vi "תפריט מוכן.vi"() -> ()   [LabVIEW 2013]
panel:
  out "current time":timestamp format="%<%I:%M %p\n%x>T"
  in  "Exit to opening screen":bool
  in  "Production":bool
  in  "Warehouse":bool
  in  "Order Manegmrnt":bool
  # "Fider"
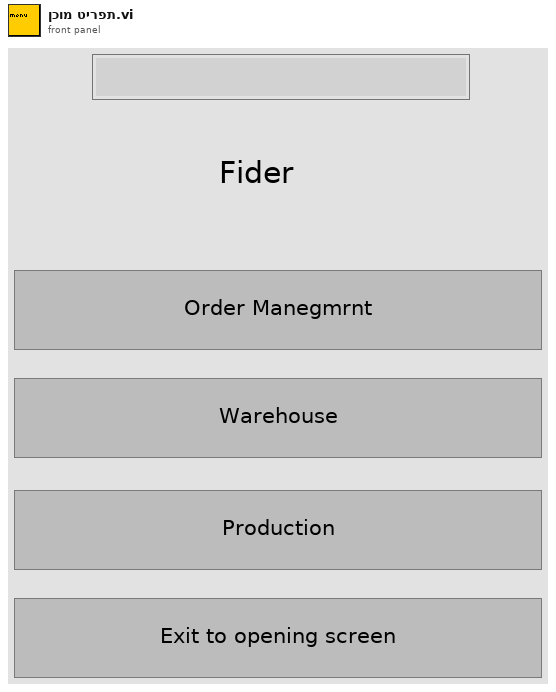
[diagram p1: front panel]
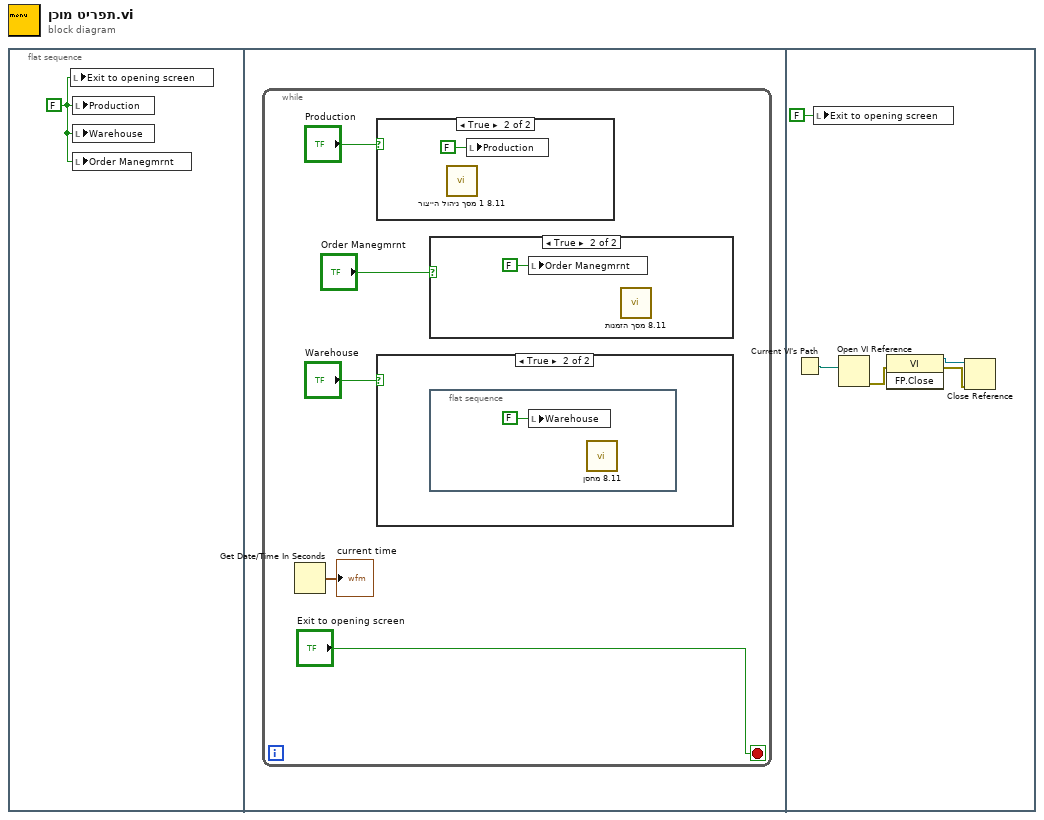
[diagram p0: block diagram]
diagram:
  n1 = flat-sequence {
    frame #0 {
      w1 = FALSE ("Exit to opening screen")
      n2 = local write "Exit to opening screen"(w1) -> ()
      n3 = local write "Production"(w1) -> ()
      n4 = local write "Warehouse"(w1) -> ()
      n5 = local write "Order Manegmrnt"(w1) -> ()
    }
    frame #1 {
      n6 = while {
        stop <- "Exit to opening screen" stop-if-true
        n7 = Get Date/Time In Seconds() -> (seconds since 1Jan1904=→"current time":timestamp)
        n8 = case shown="True" "Production" {
          frame False {
          }
          frame True {
            n9 = call "מסך ניהול הייצור 1 8.11.vi"() -> ()  [unwired: 1 in]
            n10 = local write "Production"(FALSE ("Production")) -> ()
          }
        }
        n11 = case shown="True" "Warehouse" {
          frame False {
          }
          frame True {
            n12 = flat-sequence {
              frame #0 {
                n13 = local write "Warehouse"(FALSE ("Warehouse")) -> ()
                n14 = call "מחסן 8.11.vi"() -> ()  [unwired: 1 in]
              }
            }
          }
        }
        n15 = case shown="True" "Order Manegmrnt" {
          frame False {
          }
          frame True {
            n16 = local write "Order Manegmrnt"(FALSE ("Order Manegmrnt")) -> ()
            n17 = call "מסך הזמנות 8.11.vi"() -> ()  [unwired: 1 in]
          }
        }
      }
    }
    frame #2 {
      n18 = Current VI's Path() -> (path=w13:path)
      n19 = local write "Exit to opening screen"(FALSE ("Exit to opening screen")) -> ()
      n20 = Open VI Reference(vi path=w13) -> (error out=w12:errorcluster)  [unwired: 5 in, 1 out]
      n21 = invoke class="VI" method="FP.Close"(error in=w12) -> (reference out=w10:refnum<vi>, error out=w11:errorcluster)  [unwired: 2 in, 1 out]
      n22 = Close Reference(reference=w10, error in (no error)=w11) -> ()  [unwired: 1 out]
    }
  }
